vi "Neocera21 Ramp.vi"(8 "error in (no error)":errorcluster, 11 "GPIB Adress":i16=15) -> (0 "error out":errorcluster, 2 "data string":string, 3 "?":dbl format="%.2f")   [LabVIEW 2015]
panel:
  in  "Rate, K/min":dbl=5.0 format="%.2f"
  in  "Target Temperature, K":dbl=50.0 format="%.2f"
  in  "Channel":i32=1
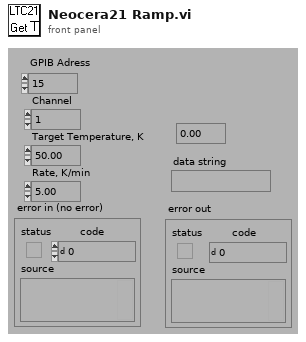
[diagram p1: front panel]
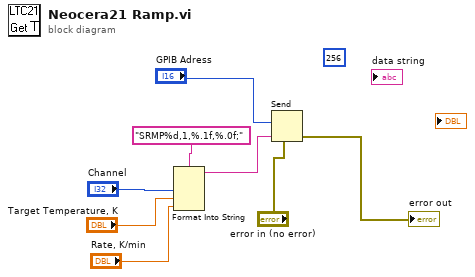
[diagram p0: block diagram]
diagram:
  (unwired) 256 ("count")
  n1 = Format Into String(format string="SRMP%d,1,%.1f,%.0f;" ("data string"), "Channel", "Target Temperature, K", "Rate, K/min") -> (resulting string=w4:string)  [unwired: 2 in, 1 out]
  n2 = Send(2:"GPIB Adress", 4:"error in (no error)", 5:w4) -> (8:→"error out":errorcluster)  [unwired: 2 in, 2 out]
